vi "RunningAverage-GetChannelRefs.vi"(8 "Error in":errorcluster, 9 "Enabled?":bool, 11 "Device Ref in":T3 format="%.0x") -> (0 "Error out":errorcluster, 1 "Parameter Block Data Refs":T1[](array[typedef]) {"Data Reference" format="%.0x"}, 2 "Result Ch Data Refs":T2[](array[typedef]) format="%.0x", 3 "Device Ref out":T3=18446744073709551615 format="%.0x")   [LabVIEW 2015, in "Waveform-Processing-Custom-Device Shared.lvlib" / "Running Average.lvlib"]
uses:
  Running Average.lvlib
  <vilib>/NI Veristand/Custom Device API/Custom Device Item Ref.ctl
  Built/Waveform-Processing-Custom-Device/Waveform-Processing-Custom-Device Engine Windows.llb/Data Reference.ctl
  <vilib>/NI Veristand/Custom Device API/Block Data Reference.ctl
  <vilib>/NI Veristand/Custom Device API/Data Access Type.ctl
  Constants.vi
  <vilib>/NI Veristand/Custom Device API/Get Item Property (Dependent Node Pointer).vi
  <vilib>/NI Veristand/Custom Device Tools/Custom Device Utility Library/NI VeriStand - Search for Item by GUID.vi
  System Explorer/Waveform-Processing-Custom-Device System Explorer.lvlib
  <vilib>/NI VeriStand/Custom Device API/Custom Device API.lvlib
  Waveform-Processing-Custom-Device Shared.lvlib
  <vilib>/NI Veristand/Custom Device Tools/Custom Device Utility Library/Custom Device Utility Library.lvlib
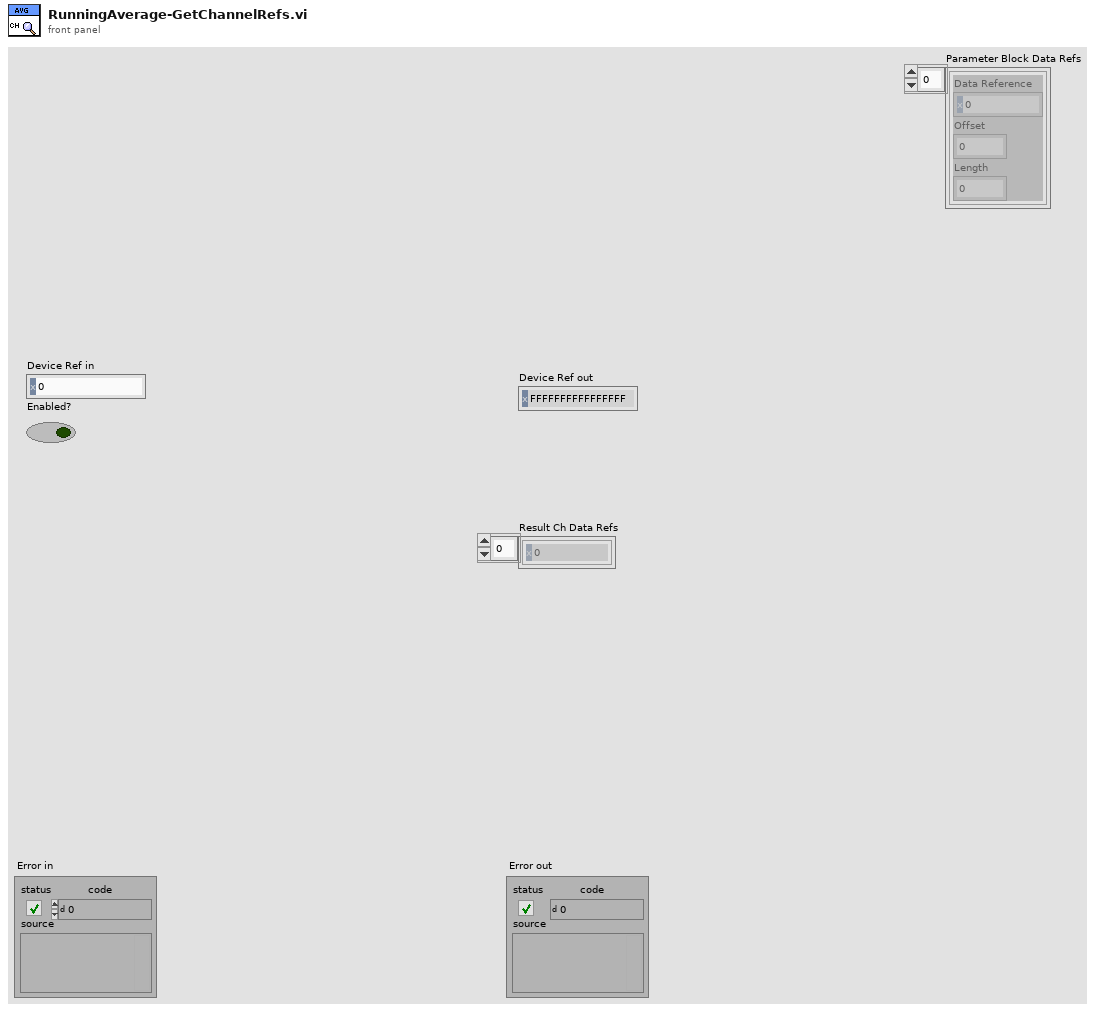
[diagram p1: front panel]
types:
  T1 = typedef "Custom Device API.lvlib/Block Data Reference.ctl" = cluster{"Data Reference":T2, "Offset":u64, "Length":u64}
  T2 = typedef "Custom Device API.lvlib/Data Reference.ctl" = i32
  T3 = typedef "Custom Device API.lvlib/Custom Device Item Ref.ctl" = u64
  T4 = typedef "Custom Device API.lvlib/Data Access Type.ctl" = enum16{"Read", "Write"}
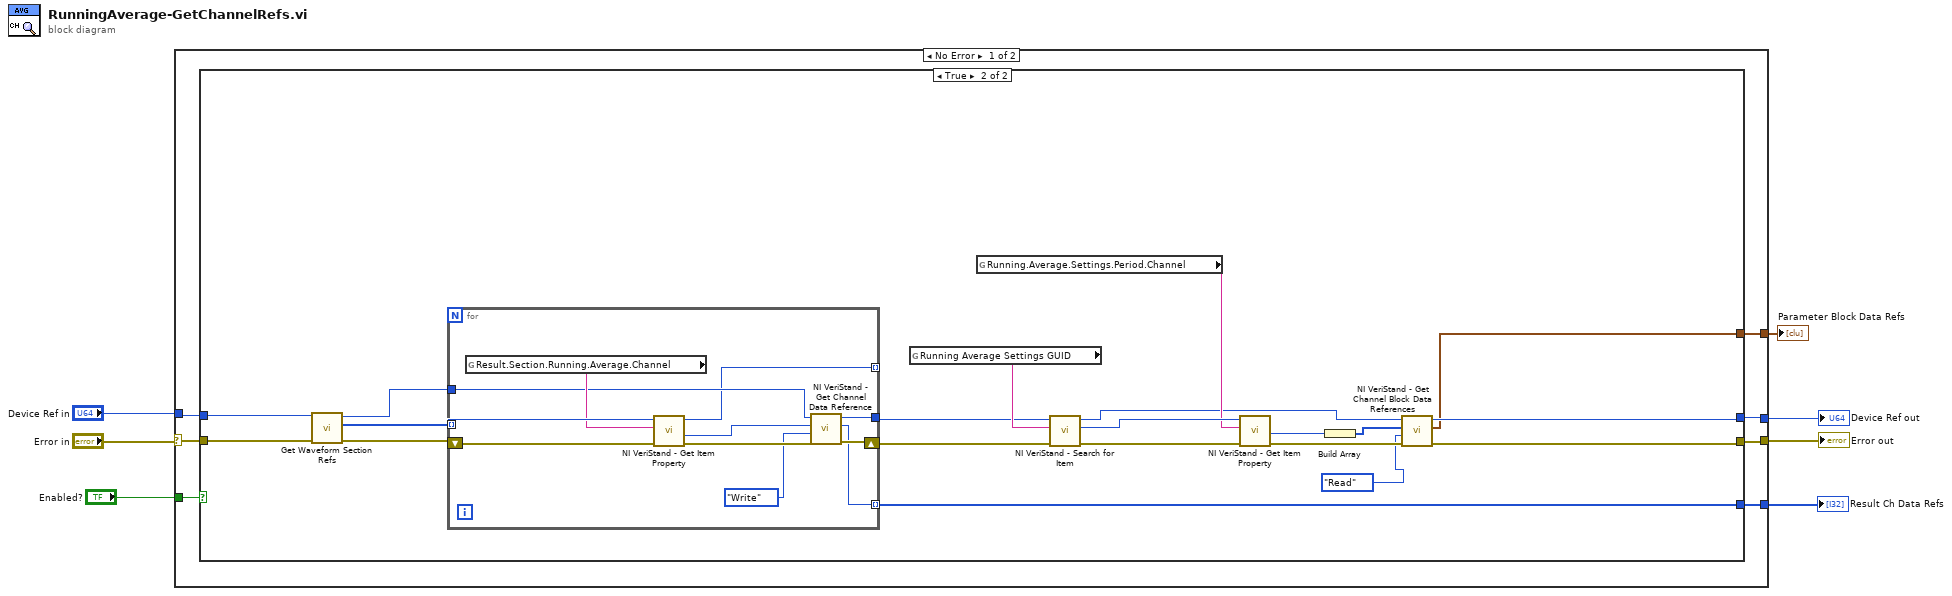
[diagram p0: block diagram]
diagram:
  n1 = case shown="No Error" "Error in" {
    selector: "Error in" -> [w14 w49]
    tunnel: [w12 w49] -> w6
    tunnel: "Device Ref in" -> [w13 w48]
    tunnel: "Enabled?" -> [w11 _]
    tunnel: [w10 w48] -> w3
    tunnel: [w9 _] -> w2
    tunnel: [w8 _] -> w1
    frame No Error {
      n2 = case shown="True" w11 {
        tunnel: w14 -> [w16 w36]
        tunnel: w13 -> [w15 w34]
        tunnel: [w16 w19] -> w12
        tunnel: [w15 w18] -> w10
        tunnel: [_ w31] -> w9
        tunnel: [_ w17] -> w8
        frame False {
        }
        frame True {
          n3 = call "Get Waveform Section Refs.vi"("Error in"=w36, "Device Ref in"=w34) -> ("Error out"=w35:errorcluster, "Result Section Refs"=w33:T3[], "Device Ref out"=w32:T3)  [unwired: 7 in]
          n4 = for {
            tunnel: w33 -> [w46] mode=indexing
            shift-right: [w43] -> w30
            shift-left: w35 -> [w47]
            tunnel: w32 -> [w41]
            tunnel: [w39] -> w28
            tunnel: [w38] -> w31 mode=indexing
            tunnel: [w37] -> _ mode=indexing
            n5 = global read "Constants.vi" "Result.Section.Running.Average.Channel"() -> (w45:string)
            n6 = call-poly <vilib>:"NI VeriStand - Get Item Property.vi"("error in (no error)"=w47, "Property Name"=w45, "Item Ref in"=w46) -> ("error out"=w44:errorcluster, "Dependent Node Ref"=w42:T3, "Item Ref out"=w37:T3)  [unwired: 5 in, 1 out]
            n7 = call <vilib>:"NI VeriStand - Get Channel Data Reference.vi"("error in (no error)"=w44, "Access"=Data_Access_Type."Write", "Channel Ref in"=w42, "Device Ref in"=w41) -> ("error out"=w43:errorcluster, "Channel Data Reference"=w38:T2, "Device Ref out"=w39:T3)  [unwired: 5 in]
          }
          n8 = global read "Constants.vi" "Running Average Settings GUID"() -> (w29:string)
          n9 = global read "Constants.vi" "Running.Average.Settings.Period.Channel"() -> (w25:string)
          n10 = call-poly <vilib>:"NI VeriStand - Search for Item.vi"("error in"=w30, "Item GUID"=w29, "Section Ref in"=w28) -> ("error out"=w27:errorcluster, "Item Ref"=w26:T3, "Section Ref out"=w20:T3)  [unwired: 5 in, 1 out]
          n11 = call-poly <vilib>:"NI VeriStand - Get Item Property.vi"("error in (no error)"=w27, "Property Name"=w25, "Item Ref in"=w26) -> ("error out"=w23:errorcluster, "Dependent Node Ref"=w24:T3)  [unwired: 5 in, 2 out]
          n12 = Build Array(w24) -> (w22:T3[])
          n13 = call <vilib>:"NI VeriStand - Get Channel Block Data References.vi"("error in (no error)"=w23, "Access"=Data_Access_Type."Read", "Channel Refs"=w22, "Device Ref in"=w20) -> ("error out"=w19:errorcluster, "Block Data Refs"=w17:T1[], "Device Ref out"=w18:T3)  [unwired: 4 in, 1 out]
        }
      }
    }
    frame Error {
    }
  }
  "Error out" <- w6
  "Device Ref out" <- w3
  "Result Ch Data Refs" <- w2
  "Parameter Block Data Refs" <- w1
